vi "plot.vi"(10 "Game Parameters":T1, 11 "Arrays and Heights":T2={"Score Array"=[], "Lowest high score"=0.0, "Score"=0.0, "Ceiling"=0.0, "Floor"=0.0, "Ceiling Array"=[], "Floor array"=[], "Helicopter height"=0.0, "Helicopter array"=[], "Fuel"=0.0, "Fuel array"=[], "fuel counter"=0, "obstacle counter"=0, "Obstacle array"=[], "helicopter v_0"=0.0, "helicopter a_0"=0.0, "Obstacle height"=300.0}) -> (3 "Waveform Chart":waveform(dbl)[](graph)=[{"t0"=timestamp(75 s since 1904-01-01), "dt"=1.0, "Y"=[90.36613236635097, 90.06036176170126, 89.42608442122003, 89.31247150775786, 88.85183588729195, 88.07425750121689, 88.69261658515198, 87.86425557558843, 88.68598594735637, 89.37218640366484, 88.87909011717896, 89.2723214289112, 89.37198808916769, 89.3075761436066, 89.59339067781413, 89.09888409349647, 89.89015333376268, 89.02148210217948, 89.47099401182557, 89.25048133248812, 89.38897358327958, 89.77746190833348, 90.53755429906346, 91.28574771023173, 90.94907051126542, 90.31859843418972, 90.86724841965984, 90.63431666280458, 91.36203841742443, 92.04622343431689, 91.2238317034208, 90.39079136550929, 89.84037866388954, 89.6430353390771, 90.19775011068187, 89.34296034585601, 88.87882107659819, 88.68974069015621, 89.40076042601159, 88.75168446743764, 87.95702372899578, 88.65736922287022, 87.90799712470135, 87.54405824486757, 87.74580039145059, 87.72021014407412, 87.91110658053051, 88.72125981331965, 88.50217712958094, 88.66901306015122, 88.44710332072938, 89.2439046034086, 89.44541276476619, 89.49348158640845, 90.23930384605846, 90.77006534815207, 91.56141906157212, 92.1965278095345, 91.61779502995512, 91.68953912575036, 91.7353123580429, 91.13420107041388, 91.29336740149286, 91.62246065547052, 92.32580838508346, 92.94681638984402, 93.63800419438708, 94.43512822801334, 95.09729030042807, 94.89218320830427, 95.29402122869416, 95.18981755244249, 94.53360430397686, 94.27656624709857, 94.95521955315563, 95.75593296599362, 95.13068608073014, 95.87345050233536, 96.41159434256669, 97.01259955208491, 96.59292222657096, 95.89637511486526, 96.58985501237102, 97.18611274172392, 97.70234591984999, 97.33615669802494, 96.72130798541049, 97.44479281384942, 97.84458360370694, 96.99411772170845, 97.83904016371078, 98.54327276615516, 98.84951280333539, 99.26520954670279, 99.7106233231448, 98.89367163173466, 98.55486364541227, 98.33140165697876, 97.47445939153363, 96.91169513152757, 96.77239204274291]}, {"t0"=timestamp(0 s since 1904-01-01), "dt"=1.0, "Y"=[50.0, 50.0, 50.0, 50.0, 50.0, 50.0, 50.0, 50.0, 50.0, 50.0, 50.0, 50.0, 50.0, 50.0, 50.0, 50.0, 50.0, 50.0, 50.0, 50.0, 50.0, 50.0, 50.0, 50.0, 50.0, 50.0, 50.0, 50.0, 50.0, 50.0, 50.0, 50.0, 50.0, 50.0, 50.0, 50.0, 50.0, 49.963212500000004, 49.901900000000005, 49.81606250000001, 49.70570000000001, 49.57081250000001, 49.41140000000001, 49.22746250000001, 49.01900000000001, 48.78601250000001, 48.528500000000015, 48.246462500000014, 47.939900000000016, 47.60881250000002, 47.25320000000002, 46.873062500000024, 46.47777500000002, 46.07358750000002, 45.66675000000002, 45.26351250000002, 44.87012500000002, 44.49283750000002, 44.13790000000002, 43.81156250000002, 43.52007500000002, 43.269687500000025, 43.066650000000024, 42.917212500000026, 42.827625000000026, 42.804137500000024, 42.85300000000002, 42.98046250000002, 43.192490909090935, 43.48605492424245, 43.861154545454575, 44.3177897727273, 44.85596060606064, 45.475667045454585, 46.176909090909135, 46.95968674242429, 47.82400000000005, 48.76984886363641, 49.79723333333339, 50.90615340909097, 52.096609090909155, 53.368600378787946, 54.72212727272734, 56.15718977272734, 57.67378787878795, 59.26254659090916, 60.91721590909098, 62.6315458333334, 64.39928636363643, 66.21418750000008, 68.06999924242433, 69.96047159090918, 71.87935454545463, 73.8203981060607, 75.77735227272736, 77.74396704545464, 79.7139924242425, 81.68117840909099, 83.63927500000008, 85.58203219696978, 87.50320000000009]}, {"t0"=timestamp(75 s since 1904-01-01), "dt"=1.0, "Y"=[5.832101008474922, 5.159278583421013, 5.801309156356126, 6.28595492791603, 6.165150175868025, 5.391838078029318, 5.660821421593425, 6.290693171535654, 5.486359312466074, 4.980595454428121, 5.743102722515479, 5.30778379381289, 5.55585812403333, 4.705780686732893, 5.2333896609954405, 4.963823736280907, 5.822464417498429, 6.642853398607047, 6.668353285980142, 6.089309556691314, 6.609858622855841, 5.982411212743665, 5.438514421617222, 6.263955715844029, 5.531193565870151, 5.801494600625852, 5.566031242846543, 5.115602472848708, 4.8481344780389595, 5.442184030722513, 5.149905285075606, 5.323279727659692, 5.065894282439003, 5.104924163660315, 4.891177011196872, 4.93812604547638, 5.067990838692791, 4.41324137869173, 3.5767367766417517, 2.792679923924744, 2.4382317997087983, 2.671144146629132, 3.1776714395653554, 3.690271474648958, 3.367994065506265, 3.215178406627257, 3.569049632721444, 3.463406971992561, 3.3200051907081365, 3.725695826201605, 3.0566988241284543, 3.4748166261830487, 2.879357702129107, 3.258851993085851, 2.522144166423153, 3.1542111118236003, 3.5230799629696405, 3.9745896259951596, 4.195366575820299, 4.883766157691795, 4.662673212944459, 5.034075317396015, 5.473994783784907, 4.699819872968005, 4.061002012703361, 3.197689491225556, 2.927623166451658, 3.7805700044544763, 3.210549827499141, 3.411153283350134, 2.6885766219340868, 3.4848113994331325, 3.8765381933384324, 3.565085003146204, 4.2186698007162295, 4.443019252189356, 4.859586669337306, 5.307331570893703, 4.60484270830926, 4.8982383059707155, 4.805761589310327, 4.454111165255858, 5.024113691840286, 4.881538126174325, 5.292346594076474, 5.233885183603672, 5.771407868577864, 5.6442442129488715, 6.45349714065848, 6.326226502898815, 5.886373600897694, 6.685385577016143, 7.325174833405951, 7.254372612866276, 7.680755742430742, 7.701210685658931, 7.8289177080882535, 8.447237862350994, 8.214394126067315, 8.955412687632835, 9.120288920602299]}, {"t0"=timestamp(75 s since 1904-01-01), "dt"=1.0, "Y"=[-150.0, -150.0, -150.0, -150.0, -150.0, -150.0, -150.0, -150.0, -150.0, -150.0, -150.0, -150.0, -150.0, -150.0, -150.0, -150.0, -150.0, -150.0, -150.0, -150.0, -150.0, -150.0, -150.0, -150.0, -150.0, -150.0, -150.0, -150.0, -150.0, -150.0, -150.0, -150.0, -150.0, -150.0, -150.0, -150.0, -150.0, -150.0, -150.0, -150.0, -150.0, -150.0, -150.0, -150.0, -150.0, -150.0, 150.0, 150.0, 150.0, 150.0, 150.0, 150.0, 150.0, 150.0, 150.0, 150.0, 38.0, 38.0, 38.0, 38.0, 38.0, 38.0, 38.0, 38.0, 38.0, 38.0, -38.0, -38.0, -38.0, -38.0, -38.0, -38.0, -38.0, -38.0, -38.0, -38.0, 5.0, 5.0, 5.0, 5.0, 5.0, 5.0, 5.0, 5.0, 5.0, 5.0, -5.0, -5.0, -5.0, -5.0, -5.0, -5.0, -5.0, -5.0, -5.0, -5.0, 9.0, 9.0, 9.0, 9.0, 9.0]}])   [LabVIEW 2017]
uses:
  controls/arrays and heights.ctl
  controls/scores.ctl
  controls/game parameters.ctl
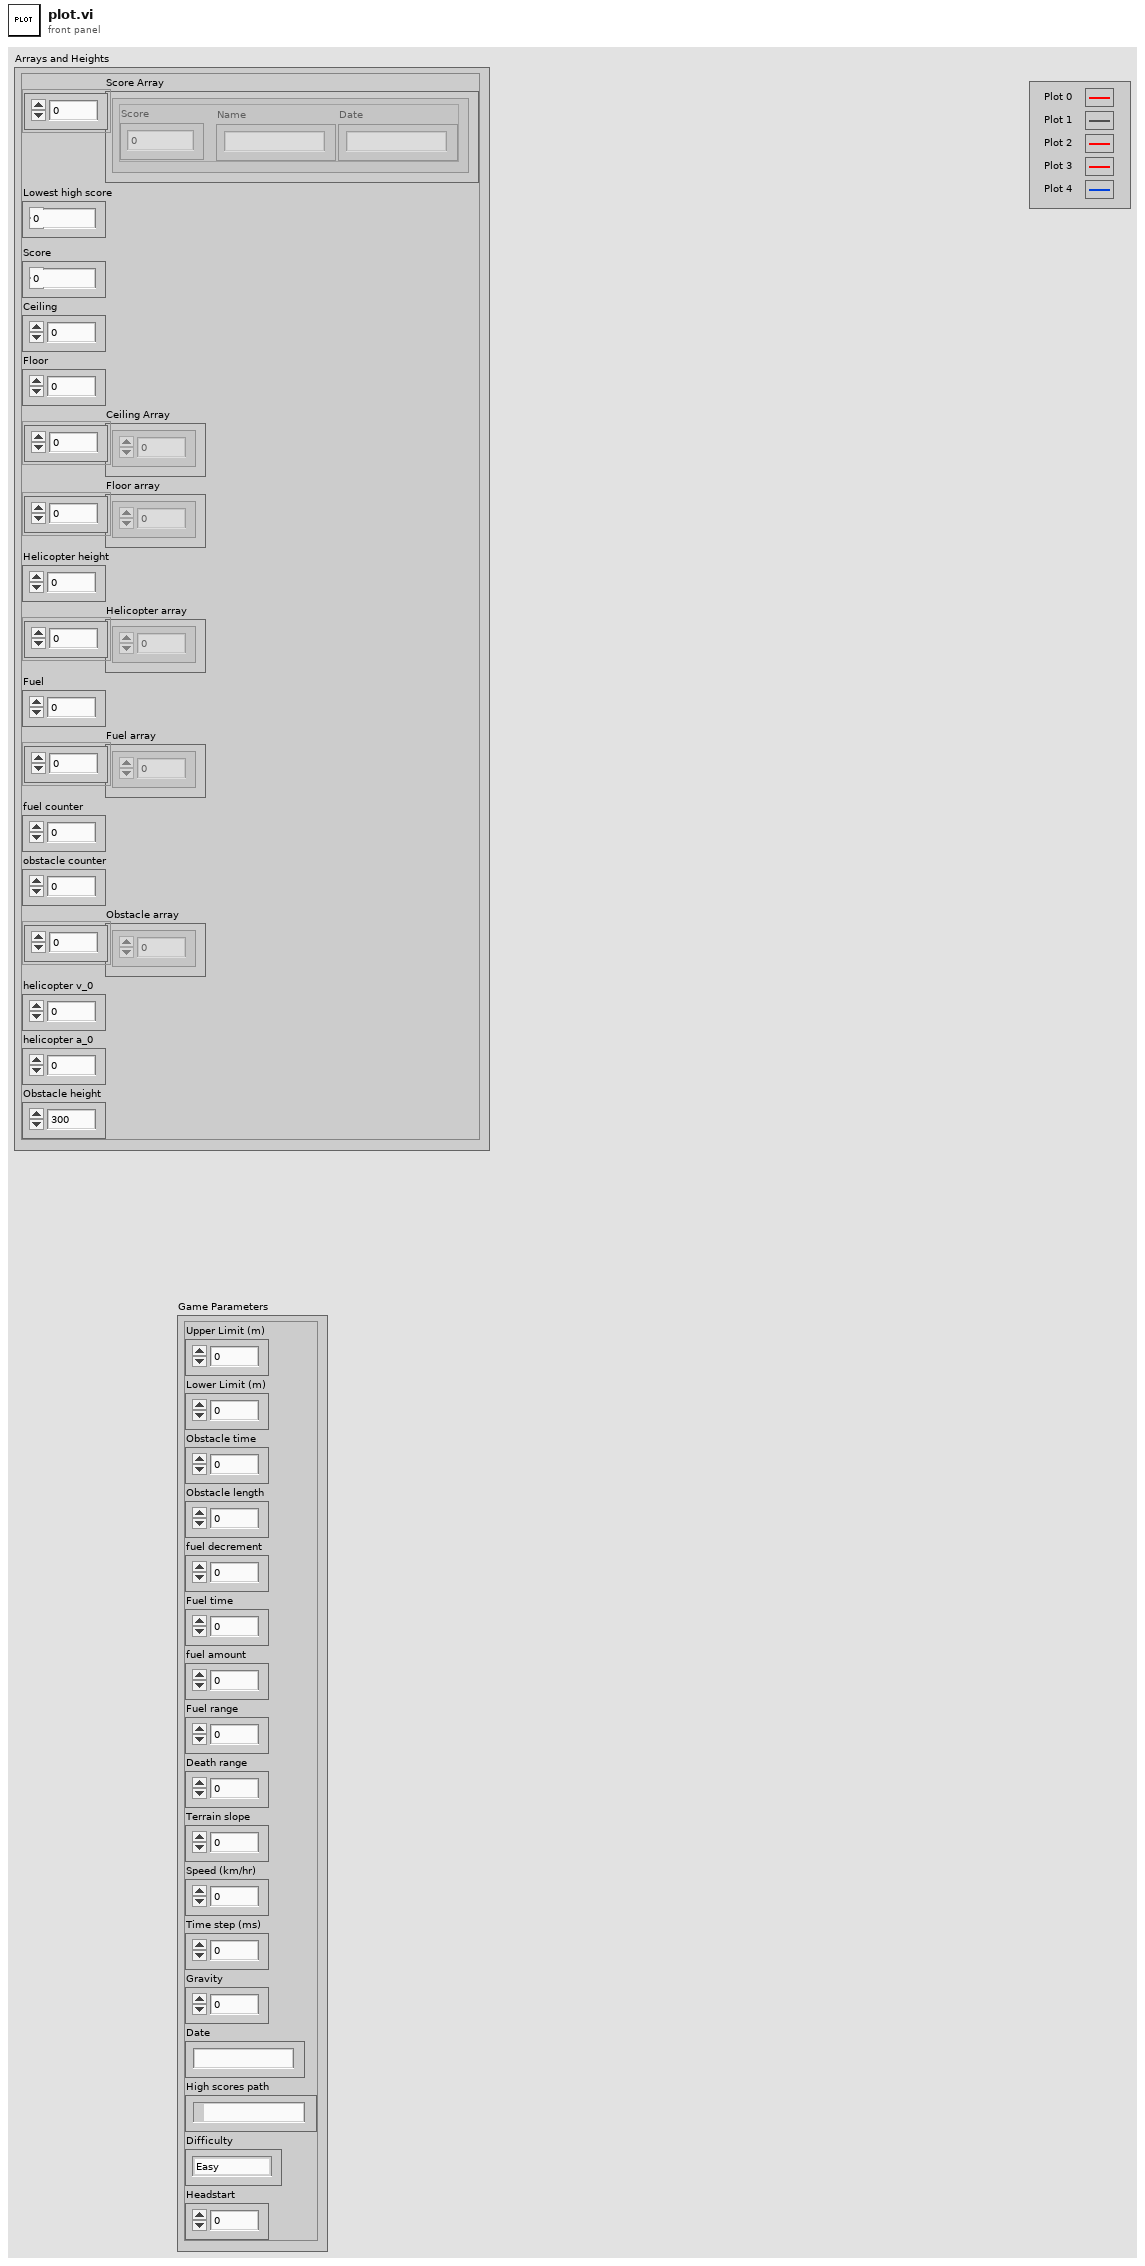
[diagram p1: front panel]
types:
  T1 = typedef "game parameters.ctl" = cluster{"Upper Limit (m)":dbl, "Lower Limit (m)":dbl, "Obstacle time":dbl, "Obstacle length":dbl, "fuel decrement":dbl, "Fuel time":dbl, "fuel amount":dbl, "Fuel range":i32, "Death range":i32, "Terrain slope":dbl, "Speed (km/hr)":dbl, "Time step (ms)":u32, "Gravity":dbl, "Date":string, "High scores path":path, "Difficulty":enum16{"Easy", "Normal", "Hard"}, "Headstart":u32}
  T2 = typedef "arrays and heights.ctl" = cluster{"Score Array":T3[], "Lowest high score":dbl, "Score":dbl, "Ceiling":dbl, "Floor":dbl, "Ceiling Array":dbl[], "Floor array":dbl[], "Helicopter height":dbl, "Helicopter array":dbl[], "Fuel":dbl, "Fuel array":dbl[], "fuel counter":i32, "obstacle counter":i32, "Obstacle array":dbl[], "helicopter v_0":dbl, "helicopter a_0":dbl, "Obstacle height":dbl}
  T3 = typedef "scores.ctl" = cluster{"Score":dbl, "Name":string, "Date":string}
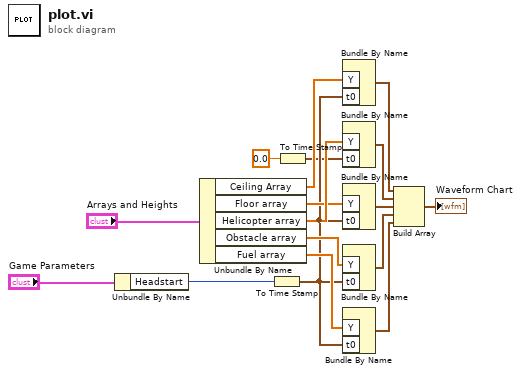
[diagram p0: block diagram]
diagram:
  n1 = Unbundle By Name("Game Parameters") -> ("Headstart"=w10:u32)
  n2 = Unbundle By Name("Arrays and Heights") -> ("Ceiling Array"=w12:dbl[], "Floor array"=w13:dbl[], "Helicopter array"=w14:dbl[], "Obstacle array"=w15:dbl[], "Fuel array"=w16:dbl[])
  n3 = To Time Stamp(1:w10) -> (0:w7:timestamp)
  n4 = To Time Stamp(1:0.0 ("number")) -> (0:w1:timestamp)
  n5 = Bundle By Name("Y"=w12, "t0"=w7) -> (w4:waveform(dbl))  [unwired: 1 in]
  n6 = Bundle By Name("Y"=w14, "t0"=w1) -> (w3:waveform(dbl))  [unwired: 1 in]
  n7 = Bundle By Name("Y"=w13, "t0"=w7) -> (w2:waveform(dbl))  [unwired: 1 in]
  n8 = Bundle By Name("Y"=w15, "t0"=w7) -> (w6:waveform(dbl))  [unwired: 1 in]
  n9 = Bundle By Name("Y"=w16, "t0"=w7) -> (w8:waveform(dbl))  [unwired: 1 in]
  n10 = Build Array(w4, w3, w2, w6, w8) -> (→"Waveform Chart":waveform(dbl)[])
